vi "Create Build Specification.vi"(8 "error in":errorcluster, 10 "measurement service name":string, 11 "project in":refnum<vi>) -> (0 "error out":errorcluster, 3 "project out":refnum<vi>)   [LabVIEW 2021, in "MeasurementService Editor.lvlib"]
uses:
  MeasurementService Editor.lvlib
  <vilib>/AppBuilder/AB_API/common/AB_API Primary Exclusions.ctl
  <vilib>/AppBuilder/AB_Source_Property_WindowRunTimePosition.ctl
  NI_AB_API_EXE_Extensions/NI_AB_API_EXE_Extensions.lvclass
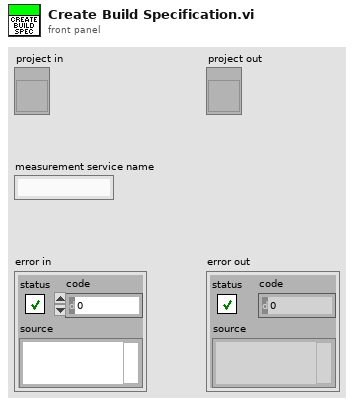
[diagram p1: front panel]
types:
  T1 = typedef "AB_Source_Property_WindowRunTimePosition.ctl" = enum16{"Unchanged", "Centered", "Maximized", "Minimized"}
  T2 = typedef "AB_API Primary Exclusions.ctl" = cluster{"Disconnect type definitions":bool, "Remove unused polymorphic VI instances":bool, "Remove unused members of project libraries":bool, "Modify project library file after removing unused members":bool}
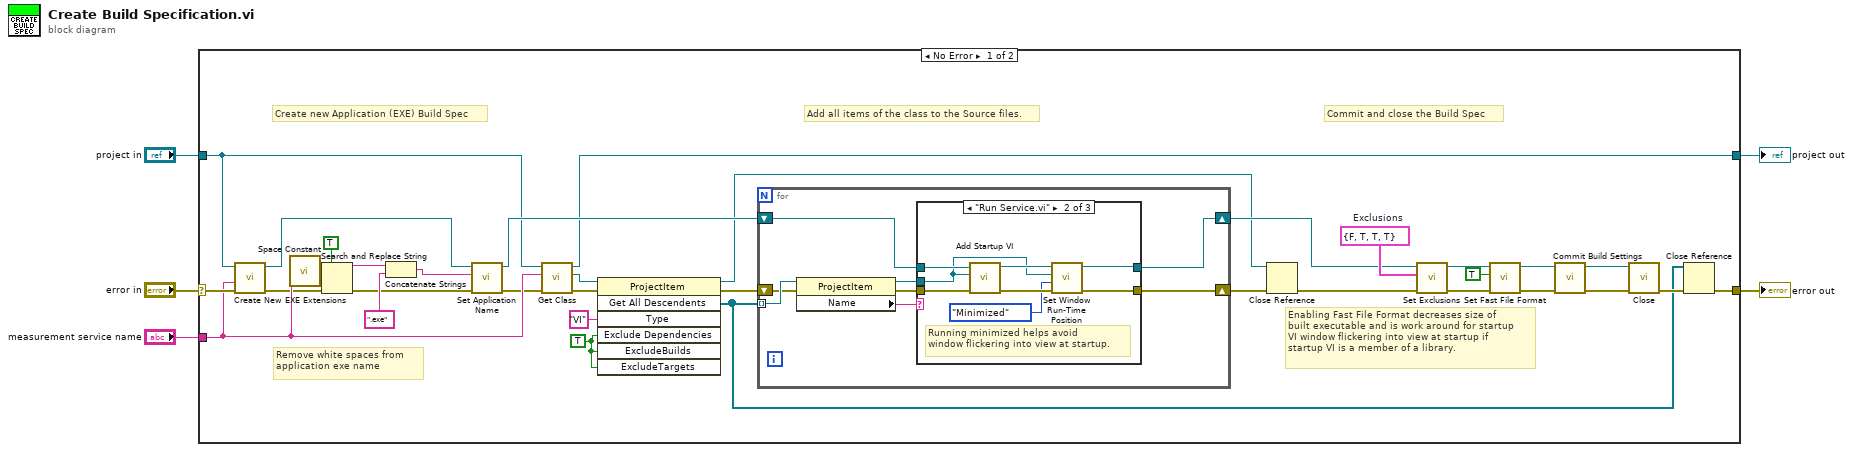
[diagram p0: block diagram]
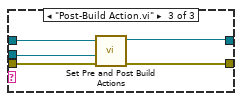
[diagram p3: hidden frame]
diagram:
  n1 = case shown="No Error" "error in" {
    selector: "error in" -> [w39 w64]
    tunnel: "project in" -> [w14 w63]
    tunnel: "measurement service name" -> [w28 _]
    tunnel: [w23 w64] -> w4
    tunnel: [w13 w63] -> w1
    frame No Error {
      w11 = TRUE ("ExcludeDependencies")
      w29 = T2 {"Disconnect type definitions"=FALSE, "Remove unused polymorphic VI instances"=TRUE, "Remove unused members of project libraries"=TRUE, "Modify project library file after removing unused members"=TRUE}  # Exclusions
      # "Enabling Fast File Format decreases size of\nbuilt executable and is work around for startup\nVI window flickering into view at startup if\nstartup VI is a member of a library."
      # "Remove white spaces from application exe name"
      # "Create new Application (EXE) Build Spec"
      # "Commit and close the Build Spec"
      # "Add all items of the class to the Source files."
      n2 = call "Create New EXE Extensions.vi"("error in (no error)"=w39, "Build specification name"=w28, "Project Refnum"=w14) -> ("error out"=w20:errorcluster, "NI_AB_API_Build out"=w21:refnum<class "NI_AB_API_EXE_Extensions.lvclass">)  [unwired: 7 in]
      n3 = call <vilib>:"Space Constant.vi"() -> ("String"=w37:string)
      n4 = Search and Replace String(replace all?=TRUE ("replace all? (F)"), input string=w28, search string=w37, error in=w20) -> (result string=w36:string, error out=w32:errorcluster)  [unwired: 4 in, 2 out]
      n5 = Concatenate Strings(w36, ".exe" ("string")) -> (w34:string)
      n6 = call-dynamic "Set Application Name.vi"("error in (no error)"=w32, "Application file name"=w34, "EXE in"=w21) -> ("error out"=w25:errorcluster, "EXE out"=w33:refnum<class "NI_AB_API_EXE_Extensions.lvclass">)  [unwired: 7 in]
      n7 = call "Get Class.vi"("error in (no error)"=w25, "class name"=w28, "project in"=w14) -> ("error out"=w27:errorcluster, "class item"=w26:refnum<vi>, "project out"=w13:refnum<vi>)  [unwired: 5 in, 1 out]
      n8 = invoke class="ProjectItem" method="Get All Descendents"(reference=w26, error in=w27, "Type"="VI", "Exclude Dependencies"=w11, "ExcludeBuilds"=w11, "ExcludeTargets"=w11) -> (reference out=w8:refnum<vi>, error out=w22:errorcluster, "All Descendents"=w6:refnum<vi>[])  [unwired: 1 in, 4 out]
      n9 = for {
        tunnel: w6 -> [w47] mode=indexing
        shift-right: [w43] -> w10
        shift-left: w33 -> [w45]
        shift-right: [w40] -> w7
        shift-left: w22 -> [w42]
        n10 = property class="ProjectItem"(reference=w47, error in=w42) -> (reference out=w44:refnum<vi>, error out=w41:errorcluster, "Name"=w46:string)
        n11 = case shown="\"Run Service.vi\"" w46 {
          tunnel: w45 -> [w49 w57 w60]
          tunnel: w44 -> [_ w51 w58]
          tunnel: [w49 w54 w59] -> w43
          tunnel: w41 -> [w48 w56 w62]
          tunnel: [w48 w52 w61] -> w40
          frame Default {
          }
          frame "Run Service.vi" {
            # "Running minimized helps avoid\nwindow flickering into view at startup."
            n12 = call-dynamic "Add Startup VI.vi"("error in (no error)"=w56, "ProjectItem Refnum"=w51, "EXE in"=w57) -> ("error out"=w53:errorcluster, "EXE out"=w55:refnum<class "NI_AB_API_EXE_Extensions.lvclass">)  [unwired: 7 in]
            n13 = call "Set Window Run-Time Position.vi"("error in (no error)"=w53, "Window Run-Time Position"=AB_Source_Property_WindowRunTimePosition."Minimized", "ProjectItem Refnum"=w51, "NI_AB_API_EXE_Extensions in"=w55) -> ("error out"=w52:errorcluster, "NI_AB_API_EXE_Extensions out"=w54:refnum<class "NI_AB_API_EXE_Extensions.lvclass">)  [unwired: 6 in]
          }
          frame "Post-Build Action.vi" {
            n14 = call-dynamic "Set Pre and Post Build Actions.vi"("error in (no error)"=w62, "Post Build Action VI"=w58, "Build in"=w60) -> ("error out"=w61:errorcluster, "Build out"=w59:refnum<class "NI_AB_API_EXE_Extensions.lvclass">)  [unwired: 7 in]
          }
        }
      }
      n15 = Close Reference(reference=w8, error in (no error)=w7) -> (error out=w9:errorcluster)
      n16 = call-dynamic "Set Exclusions.vi"("error in (no error)"=w9, "Exclusions"=w29, "EXE in"=w10) -> ("error out"=w17:errorcluster, "EXE out"=w19:refnum<class "NI_AB_API_EXE_Extensions.lvclass">)  [unwired: 7 in]
      n17 = call "Set Fast File Format.vi"("error in (no error)"=w17, "Enable Fast File Format"=TRUE, "NI_AB_API_EXE_Extensions in"=w19) -> ("error out"=w16:errorcluster, "NI_AB_API_EXE_Extensions out"=w18:refnum<class "NI_AB_API_EXE_Extensions.lvclass">)  [unwired: 7 in]
      n18 = call-dynamic "Commit Build Settings.vi"("error in (no error)"=w16, "EXE in"=w18) -> ("error out"=w30:errorcluster, "EXE out"=w31:refnum<class "NI_AB_API_EXE_Extensions.lvclass">)  [unwired: 8 in]
      n19 = call-dynamic "Close.vi"("error in (no error)"=w30, "EXE in"=w31) -> ("error out"=w24:errorcluster)  [unwired: 9 in]
      n20 = Close Reference(reference=w6, error in (no error)=w24) -> (error out=w23:errorcluster)
    }
    frame Error {
    }
  }
  "error out" <- w4
  "project out" <- w1
